vi "Server.vi"() -> ()   [LabVIEW 2021]
panel:
  in  "Knob":dbl(knob) scale=0.0..10.0
  in  "Stop":bool
  # "HOST"
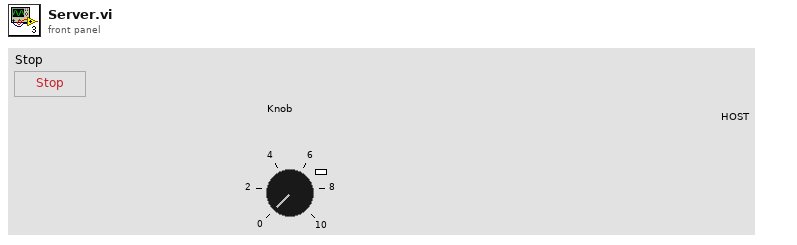
[diagram p1: front panel]
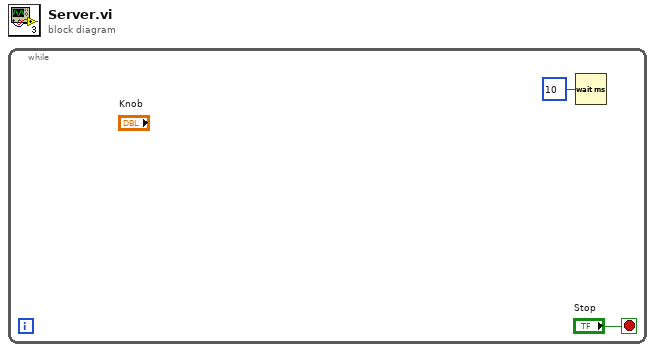
[diagram p0: block diagram]
diagram:
  n1 = while {
    stop <- "Stop" stop-if-true
    n2 = Wait (ms)(milliseconds to wait=u32 10) -> ()  [unwired: 1 out]
  }
